vi "getcurrentposition.vi"() -> ()   [LabVIEW 2013]
panel:
  in  "Distance":dbl
  in  "Set First":bool
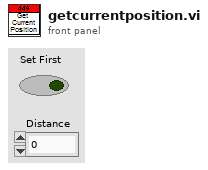
[diagram p1: front panel]
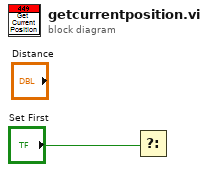
[diagram p0: block diagram]
diagram:
  n1 = Select(s="Set First") -> ()  [unwired: 2 in, 1 out]
